vi "SGUI Set Value and Uncertainty to String By Label.vi"   [LabVIEW 2020, in "varilib.lvlib"]
doc: "This VI sets '(value ± uncerainty) unit' into string control defined by control label (must be registered first by calling 'SGUI Register Controls'). The formatter also does SI prefix scaling which can be optionally disabled (mostly for unitless quantities). It automatically formats the value and uncertainty to two significant digits of uncertainty. If unit is assigned it will append it after the value and uncertainty. If no value is assigned it will assign empty string (NaN is considered as no input). It will generate error if control not found or has ivalid type but it ignores input errors (executes anyway)."
uses:
  varilib.lvlib
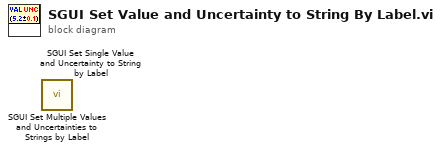
[diagram p0: block diagram]
diagram:
  n1 = call "SGUI Set Multiple Values and Uncertainties to Strings by Label.vi"() -> ()  [unwired: 14 in, 2 out]
  n2 = call "SGUI Set Single Value and Uncertainty to String by Label.vi"() -> ()  [unwired: 14 in, 2 out]
